vi "ROI-SelectionAndorOne.vi"(8 "error in (no error)":errorcluster, 9 "Global Rectangle":i32[](array[numeric]), 11 "Image In":i32[][](array[numeric])) -> (0 "error out":errorcluster, 2 "output cluster":T1, 3 "Image Out":i32[][](array[numeric]))   [LabVIEW 2011]
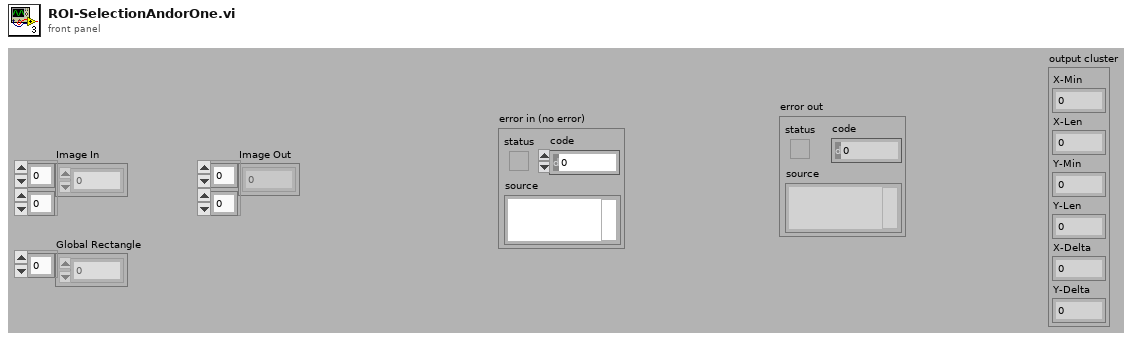
[diagram p1: front panel]
types:
  T1 = cluster{"X-Min":i32, "X-Len":i32, "Y-Min":i32, "Y-Len":i32, "X-Delta":i32, "Y-Delta ":i32}
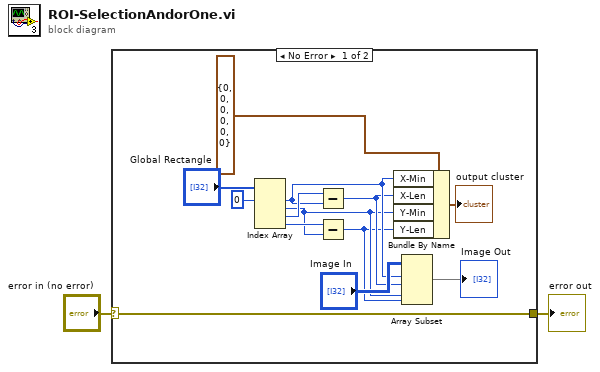
[diagram p0: block diagram]
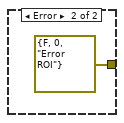
[diagram p2: hidden frame]
diagram:
  n1 = case shown="No Error" "error in (no error)" {
    selector: "error in (no error)" -> [w5 _]
    tunnel: [w5 errorcluster {"status"=FALSE, "code"=0, "source"="Error ROI"} ("error IO")] -> w1
    frame No Error {
      n2 = Index Array(array="Global Rectangle", index #1=0 ("index")) -> (element #1=w9:i32, element #2=w7:i32, element #3=w12:i32, element #4=w13:i32)  [unwired: 3 in]
      n3 = Subtract(x=w12, y=w9) -> (x-y=w8:i32)
      n4 = Subtract(x=w13, y=w7) -> (x-y=w6:i32)
      n5 = Bundle By Name(cluster=T1 {"X-Min"=0, "X-Len"=0, "Y-Min"=0, "Y-Len"=0, "X-Delta"=0, "Y-Delta "=0} ("ROI Coordinates out"), "X-Min"=w9, "X-Len"=w8, "Y-Min"=w7, "Y-Len"=w6) -> (→"output cluster":T1)
      n6 = Array Subset(array="Image In", index (row)=w9, length (row)=w8, index (col)=w7, length (col)=w6) -> (→"Image Out":i32[][])
    }
    frame Error {
    }
  }
  "error out" <- w1
